vi "move.vi"(0 "x distance":dbl, 1 "y distance":dbl, 2 "z distance":dbl, 3 "button com":bool, 6 "handle":i32, 8 "halt":refnum<vi>, 9 "device ID":refnum<k1>, 10 "velocityZ":dbl, 11 "Encoder":T1, 12 "velocityX":dbl, 13 "velocityY":dbl, 14 "X Axis":u16(ring)=2 items=["X axis", "Y axis", "Z axis", "X axis rotation", "Y axis rotation", "Z axis rotation", "U axis", "V axis"], 15 "Y Axis":u16(ring)=1 items=["X axis", "Y axis", "Z axis", "X axis rotation", "Y axis rotation", "Z axis rotation", "U axis", "V axis"], 16 "Invert":bool, 17 "Invert 2":bool=TRUE, 18 "Invert 3":bool=TRUE, 19 "Z Axis":u16(ring)=4 items=["X axis", "Y axis", "Z axis", "X axis rotation", "Y axis rotation", "Z axis rotation", "U axis", "V axis"]) -> ()   [LabVIEW 2012]
uses:
  <vilib>/Utility/inputDevices.llb/joystickAcquire.vi
  MicroDrive.dll
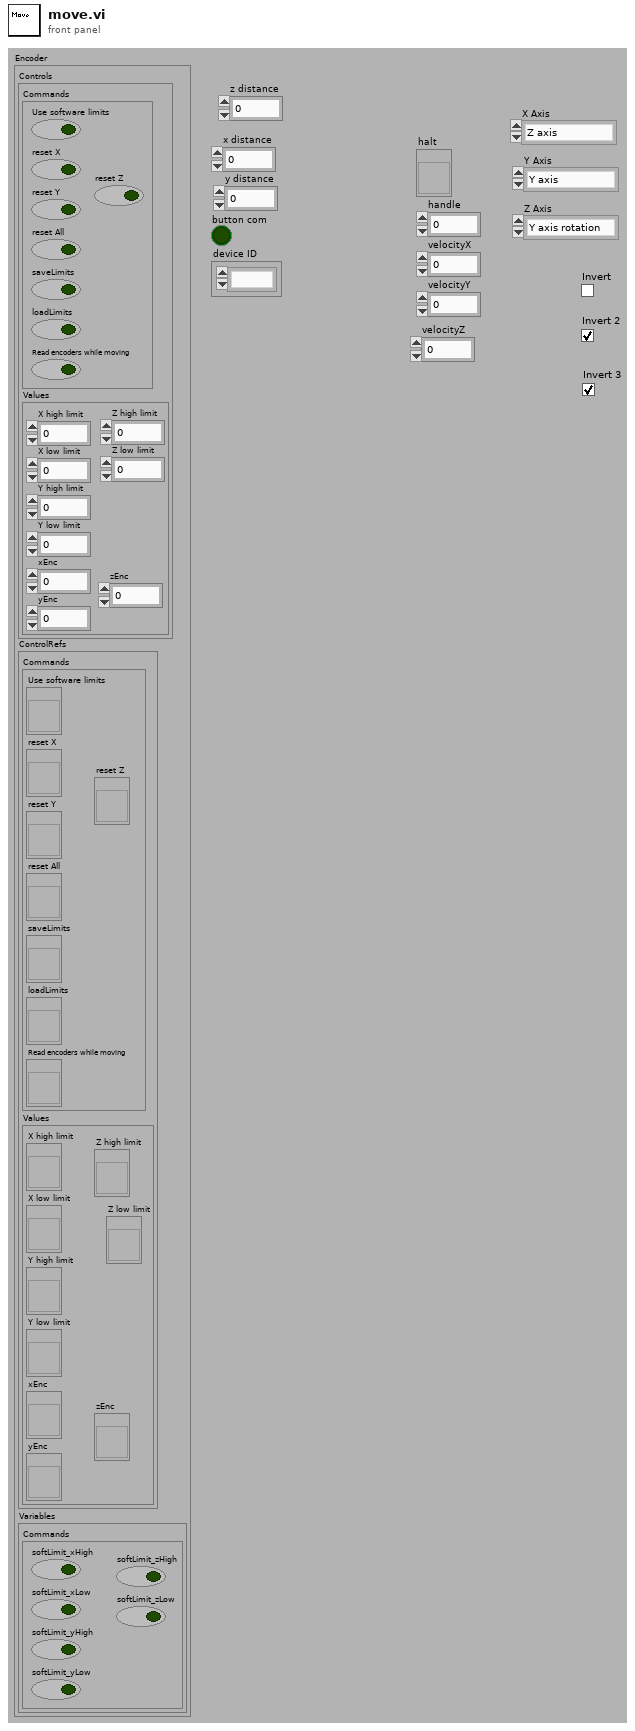
[diagram p1: front panel]
types:
  T1 = cluster{"Controls":cluster{"Commands":cluster{"Use software limits":bool, "reset X":bool, "reset Y":bool, "reset All":bool, "saveLimits":bool, "loadLimits":bool, "Read encoders while moving":bool, "reset Z":bool}, "Values":cluster{"X high limit":dbl, "X low limit":dbl, "Y high limit":dbl, "Y low limit":dbl, "xEnc":dbl, "yEnc":dbl, "Z low limit":dbl, "Z high limit":dbl, "zEnc":dbl}}, "ControlRefs":cluster{"Commands":cluster{"Use software limits":refnum<vi>, "reset X":refnum<vi>, "reset Y":refnum<vi>, "reset All":refnum<vi>, "saveLimits":refnum<vi>, "loadLimits":refnum<vi>, "Read encoders while moving":refnum<vi>, "reset Z":refnum<vi>}, "Values":cluster{"X high limit":refnum<vi>, "X low limit":refnum<vi>, "Y high limit":refnum<vi>, "Y low limit":refnum<vi>, "xEnc":refnum<vi>, "yEnc":refnum<vi>, "Z low limit":refnum<vi>, "Z high limit":refnum<vi>, "zEnc":refnum<vi>}}, "Variables":cluster{"Commands":cluster{"softLimit_xHigh":bool, "softLimit_xLow":bool, "softLimit_yHigh":bool, "softLimit_yLow":bool, "softLimit_zLow":bool, "softLimit_zHigh":bool}}}
  T2 = cluster{"xDistance":dbl, "yDistance":dbl, "xMove":bool, "yMove":bool, "zDistance":dbl, "zMove":bool}
  T3 = cluster{"Boolean array[0]":bool, "Boolean array[1]":bool, "Boolean array[2]":bool, "Boolean array[3]":bool, "Boolean array[4]":bool, "Boolean array[5]":bool, "Boolean array[6]":bool, "Boolean array[7]":bool, "Boolean array[8]":bool, "Boolean array[9]":bool, "Boolean array[10]":bool, "Boolean array[11]":bool, "Boolean array[12]":bool, "Boolean array[13]":bool, "Boolean array[14]":bool, "Boolean array[15]":bool}
  T4 = cluster{"X axis":i32, "Y axis":i32, "Z axis":i32, "X axis rotation":i32, "Y axis rotation":i32, "Z axis rotation":i32, "U axis":i32, "V axis":i32}
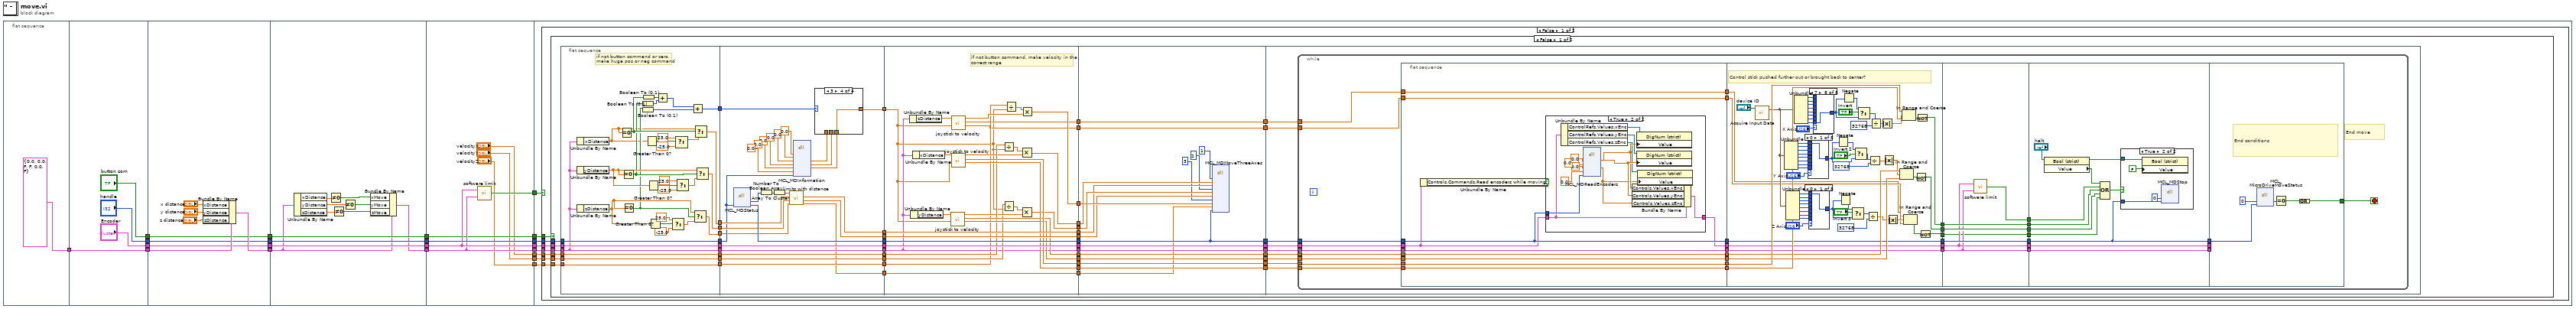
[diagram p0: block diagram]
diagram:
  n1 = flat-sequence {
    tunnel: [T2 {"xDistance"=0.0, "yDistance"=0.0, "xMove"=FALSE, "yMove"=FALSE, "zDistance"=0.0, "zMove"=FALSE}] -> w16
    tunnel: w16 -> [w26]
    tunnel: [w26] -> w15
    tunnel: ["Encoder"] -> w14
    tunnel: ["handle"] -> w13
    tunnel: ["button com"] -> w12
    tunnel: w15 -> [w34]
    tunnel: [w31] -> w21
    tunnel: w14 -> [w30]
    tunnel: w13 -> [w29]
    tunnel: w12 -> [w28]
    tunnel: [w30] -> w11
    tunnel: [w29] -> w10
    tunnel: [w28] -> w9
    tunnel: [w45] -> w7
    tunnel: [w43] -> w6
    tunnel: [w42] -> w5
    tunnel: [w44] -> w4
    tunnel: w9 -> [w44]
    tunnel: w10 -> [w45]
    tunnel: w11 -> [w43]
    tunnel: w21 -> [w38]
    tunnel: w7 -> [w53]
    tunnel: [w53] -> w20
    tunnel: w6 -> [w52]
    tunnel: [w52] -> w19
    tunnel: w5 -> [w51]
    tunnel: [w51] -> w18
    tunnel: [w50] -> w17
    tunnel: [w49] -> w8
    tunnel: w4 -> [w49]
    tunnel: ["velocityX"] -> w3
    tunnel: ["velocityY"] -> w2
    tunnel: ["velocityZ"] -> w1
    tunnel: w20 -> [w61]
    tunnel: w19 -> [w60]
    tunnel: w18 -> [w59]
    tunnel: w17 -> [w58]
    tunnel: w8 -> [w57]
    tunnel: w3 -> [w56]
    tunnel: w2 -> [w55]
    tunnel: w1 -> [w54]
    frame #0 {
    }
    frame #1 {
    }
    frame #2 {
      n2 = Bundle By Name(cluster=w34, "xDistance"="x distance", "yDistance"="y distance", "zDistance"="z distance") -> (w31:T2)
    }
    frame #3 {
      n3 = Unbundle By Name(w38) -> ("xDistance"=w41:dbl, "yDistance"=w37:dbl, "zDistance"=w36:dbl)
      n4 = Not Equal To 0?(x=w41) -> (x != 0?=w40:bool)
      n5 = Not Equal To 0?(x=w36) -> (x != 0?=w35:bool)
      n6 = Not Equal To 0?(x=w37) -> (x != 0?=w39:bool)
      n7 = Bundle By Name(cluster=w38, "xMove"=w40, "yMove"=w39, "zMove"=w35) -> (w42:T2)
    }
    frame #4 {
      n8 = call "software limit.vi"("variables"=w51, "Encoder"=w52) -> ("limited"=w50:bool)
    }
    frame #5 {
      n9 = case shown="False" w58 {
        tunnel: w57 -> [w68 _]
        tunnel: w61 -> [w67 _]
        tunnel: w60 -> [w66 _]
        tunnel: w59 -> [w65 _]
        tunnel: w56 -> [w64 _]
        tunnel: w55 -> [w63 _]
        tunnel: w54 -> [w62 _]
        frame False {
          n10 = case shown="False" w68 {
            tunnel: w67 -> [w118 w421]
            tunnel: w66 -> [w117 w420]
            tunnel: w65 -> [w112 w419]
            tunnel: w64 -> [w93 w415]
            tunnel: w63 -> [w91 w414]
            tunnel: w62 -> [w81 w413]
            frame False {
              n11 = flat-sequence {
                tunnel: w117 -> [w149]
                tunnel: w118 -> [w150]
                tunnel: [w150] -> w116
                tunnel: [w140] -> w115
                tunnel: [w139] -> w114
                tunnel: [w149] -> w113
                tunnel: w112 -> [w136]
                tunnel: [w136] -> w111
                tunnel: [w138] -> w94
                tunnel: w93 -> [w138]
                tunnel: [w137] -> w92
                tunnel: w91 -> [w137]
                tunnel: w81 -> [w129]
                tunnel: [w132] -> w80
                tunnel: [w129] -> w79
                tunnel: [w119] -> w70
                tunnel: [w175] -> w110
                tunnel: [w166] -> w108
                tunnel: [w165] -> w106
                tunnel: [w171] -> w104
                tunnel: w116 -> [w164]
                tunnel: w115 -> [w173]
                tunnel: w114 -> [w172]
                tunnel: w113 -> [w171]
                tunnel: [w170] -> w102
                tunnel: w111 -> [w170]
                tunnel: w94 -> [w169]
                tunnel: w92 -> [w168]
                tunnel: [w169] -> w90
                tunnel: [w168] -> w89
                tunnel: w80 -> [w152]
                tunnel: w79 -> [w167]
                tunnel: [w167] -> w78
                tunnel: [w151] -> w76
                tunnel: w70 -> [w157]
                tunnel: [w153] -> w69
                tunnel: w110 -> [w209]
                tunnel: [w209] -> w109
                tunnel: w108 -> [w208]
                tunnel: [w208] -> w107
                tunnel: w106 -> [w207]
                tunnel: [w207] -> w105
                tunnel: w104 -> [w206]
                tunnel: [w206] -> w103
                tunnel: w102 -> [w192]
                tunnel: [w192] -> w101
                tunnel: [w197] -> w100
                tunnel: [w203] -> w99
                tunnel: [w202] -> w98
                tunnel: [w194] -> w97
                tunnel: [w201] -> w96
                tunnel: [w200] -> w95
                tunnel: w90 -> [w199]
                tunnel: w89 -> [w193]
                tunnel: w78 -> [w186]
                tunnel: [w189] -> w77
                tunnel: w76 -> [w185]
                tunnel: [w185] -> w75
                tunnel: [w184] -> w73
                tunnel: [w183] -> w71
                tunnel: w69 -> [w182]
                tunnel: [w227] -> w88
                tunnel: [w226] -> w87
                tunnel: [w225] -> w86
                tunnel: [w224] -> w85
                tunnel: [w223] -> w84
                tunnel: [w221] -> w83
                tunnel: [w222] -> w82
                tunnel: w95 -> [w224]
                tunnel: w96 -> [w225]
                tunnel: w97 -> [w217]
                tunnel: w98 -> [w226]
                tunnel: w99 -> [w227]
                tunnel: w100 -> [w218]
                tunnel: w101 -> [w222]
                tunnel: w103 -> [w223]
                tunnel: w105 -> [w214]
                tunnel: w107 -> [w215]
                tunnel: w109 -> [w221]
                tunnel: w77 -> [w216]
                tunnel: w75 -> [w213]
                tunnel: [w220] -> w74
                tunnel: w73 -> [w220]
                tunnel: [w219] -> w72
                tunnel: w71 -> [w219]
                tunnel: w88 -> [w236]
                tunnel: w87 -> [w235]
                tunnel: w86 -> [w234]
                tunnel: w85 -> [w233]
                tunnel: w84 -> [w232]
                tunnel: w83 -> [w231]
                tunnel: w82 -> [w230]
                tunnel: w74 -> [w229]
                tunnel: w72 -> [w228]
                frame #0 {
                  # "if not button command or zero,\nmake huge pos or neg command"
                  n12 = Unbundle By Name(w136) -> ("yDistance"=w127:dbl)
                  n13 = Unbundle By Name(w136) -> ("xDistance"=w120:dbl)
                  n14 = Unbundle By Name(w136) -> ("zDistance"=w130:dbl)
                  n15 = Equal To 0?(x=w120) -> (x = 0?=w128:bool)
                  n16 = Equal To 0?(x=w127) -> (x = 0?=w122:bool)
                  n17 = Equal To 0?(x=w130) -> (x = 0?=w121:bool)
                  n18 = Boolean To (0,1)(Boolean=w122) -> (0, 1=w125:i16)
                  n19 = Boolean To (0,1)(Boolean=w121) -> (0, 1=w124:i16)
                  n20 = Boolean To (0,1)(Boolean=w128) -> (0, 1=w126:i16)
                  n21 = Greater Than 0?(x=w120) -> (x > 0?=w147:bool)
                  n22 = Greater Than 0?(x=w127) -> (x > 0?=w143:bool)
                  n23 = Greater Than 0?(x=w130) -> (x > 0?=w135:bool)
                  n24 = Add(x=w126, y=w125) -> (x+y=w123:i16)
                  n25 = Select(t=25.0, s=w135, f=-25.0) -> (s? t:f=w131:dbl)
                  n26 = Select(t=25.0, s=w147, f=-25.0) -> (s? t:f=w148:dbl)
                  n27 = Select(t=25.0, s=w143, f=-25.0) -> (s? t:f=w144:dbl)
                  n28 = Add(x=w123, y=w124) -> (x+y=w119:i16)
                  n29 = Select(t=w130, s=w121, f=w131) -> (s? t:f=w132:dbl)
                  n30 = Select(t=w120, s=w128, f=w148) -> (s? t:f=w140:dbl)
                  n31 = Select(t=w127, s=w122, f=w144) -> (s? t:f=w139:dbl)
                }
                frame #1 {
                  n32 = dll-call lib="C:/Users/Labview/Desktop/SRR/MicroDrive_x64/Labview Examples/MicroDrive.dll" fn="MCL_MDStatus"("handle"=w164) -> ("status"=w177:u16, "handle"=w175:i32)  [unwired: 3 in, 4 out]
                  n33 = Number To Boolean Array(number=w177) -> (Boolean array=w176:bool[])
                  n34 = Array To Cluster(array=w176) -> (cluster=w174:T3)
                  n35 = call "limits with distance.vi"("distanceM3"=w152, "distanceM2"=w172, "distanceM1"=w173, "cluster"=w174) -> ("M3 Distance"=w151:dbl, "M2 Distance"=w165:dbl, "M1 Distance"=w166:dbl)  [unwired: 1 in, 4 out]
                  n36 = dll-call lib="C:/Users/Labview/Desktop/SRR/MicroDrive_x64/Labview Examples/MicroDrive.dll" fn="MCL_MDInformation"("encoderResolution"=0.0 ("t"), "stepSize"=0.0 ("t"), "maxVelocity"=0.0 ("t"), "maxVelocityTwoAxis"=0.0 ("t"), "maxVelocityThreeAxis"=0.0 ("t"), "minVelocity"=0.0 ("t"), "handle"=w164) -> ("maxVelocity"=w156:dbl, "maxVelocityTwoAxis"=w155:dbl, "maxVelocityThreeAxis"=w154:dbl)  [unwired: 4 in, 6 out]
                  n37 = case shown="3" w157 {
                    tunnel: w156 -> [w178 w179 _ _]
                    tunnel: w155 -> [_ _ w180 _]
                    tunnel: w154 -> [_ _ _ w181]
                    tunnel: [w178 w179 w180 w181] -> w153
                    frame 0, Default {
                    }
                    frame 1 {
                    }
                    frame 2 {
                    }
                    frame 3 {
                    }
                  }
                }
                frame #2 {
                  # "if not button command, make velocity in the\ncorrect range"
                  n38 = Unbundle By Name(w192) -> ("zDistance"=w191:dbl)
                  n39 = Unbundle By Name(w192) -> ("yDistance"=w205:dbl)
                  n40 = Unbundle By Name(w192) -> ("xDistance"=w204:dbl)
                  n41 = call "joystick to velocity.vi"("max velocity"=w182, "joystick main"=w205) -> ("lower bound"=w200:dbl, "upper bound"=w201:dbl, "Velocity"=w195:dbl)  [unwired: 2 in, 5 out]
                  n42 = call "joystick to velocity.vi"("max velocity"=w182, "joystick main"=w191) -> ("lower bound"=w183:dbl, "upper bound"=w184:dbl, "Velocity"=w187:dbl)  [unwired: 2 in, 5 out]
                  n43 = call "joystick to velocity.vi"("max velocity"=w182, "joystick main"=w204) -> ("lower bound"=w202:dbl, "upper bound"=w203:dbl, "Velocity"=w198:dbl)  [unwired: 2 in, 5 out]
                  n44 = Divide(x=w199, y=w182) -> (x/y=w190:dbl)
                  n45 = Divide(x=w193, y=w182) -> (x/y=w196:dbl)
                  n46 = Divide(x=w186, y=w182) -> (x/y=w188:dbl)
                  n47 = Multiply(x=w190, y=w198) -> (x*y=w197:dbl)
                  n48 = Multiply(x=w196, y=w195) -> (x*y=w194:dbl)
                  n49 = Multiply(x=w188, y=w187) -> (x*y=w189:dbl)
                }
                frame #3 {
                  n50 = dll-call lib="C:/Users/Labview/Desktop/SRR/MicroDrive_x64/Labview Examples/MicroDrive.dll" fn="MCL_MDMoveThreeAxes"("axis1"=1 ("rounding-X"), "Velocity-1"=w218, "distance-1"=w215, "axis2"=2 ("rounding-X"), "Velocity-2"=w217, "distance-2"=w214, "axis3"=3 ("rounding-X"), "Velocity-3"=w216, "Distance-3"=w213, "handle"=w221) -> ()  [unwired: 14 in, 2 out]
                }
                frame #4 {
                  n51 = while {
                    tunnel: w236 -> [w270]
                    tunnel: w235 -> [w269]
                    tunnel: w234 -> [w268]
                    tunnel: w233 -> [w267]
                    tunnel: w232 -> [w266]
                    tunnel: w231 -> [w265]
                    tunnel: w230 -> [w262]
                    tunnel: w229 -> [w240]
                    tunnel: w228 -> [w238]
                    stop <- w271 stop-if-true
                    # "End move"
                    n52 = flat-sequence {
                      tunnel: w262 -> [w276]
                      tunnel: w265 -> [w278]
                      tunnel: w266 -> [w275]
                      tunnel: w267 -> [w279]
                      tunnel: w268 -> [w280]
                      tunnel: w269 -> [w281]
                      tunnel: w270 -> [w282]
                      tunnel: [w282] -> w249
                      tunnel: [w281] -> w248
                      tunnel: [w280] -> w247
                      tunnel: [w279] -> w246
                      tunnel: [w277] -> w245
                      tunnel: [w278] -> w244
                      tunnel: [w276] -> w243
                      tunnel: w240 -> [w273]
                      tunnel: [w273] -> w239
                      tunnel: w238 -> [w272]
                      tunnel: [w272] -> w237
                      tunnel: [w321] -> w260
                      tunnel: [w324] -> w258
                      tunnel: [w339] -> w256
                      tunnel: [w322] -> w254
                      tunnel: [w320] -> w252
                      tunnel: w249 -> [w342]
                      tunnel: w248 -> [w341]
                      tunnel: w247 -> [w329]
                      tunnel: w246 -> [w340]
                      tunnel: w245 -> [w322]
                      tunnel: w244 -> [w321]
                      tunnel: w243 -> [w320]
                      tunnel: [w307] -> w242
                      tunnel: w239 -> [w297]
                      tunnel: w237 -> [w298]
                      tunnel: w260 -> [w392]
                      tunnel: [w392] -> w259
                      tunnel: w258 -> [w391]
                      tunnel: [w391] -> w257
                      tunnel: w256 -> [w390]
                      tunnel: [w390] -> w255
                      tunnel: w254 -> [w388]
                      tunnel: [w388] -> w253
                      tunnel: w252 -> [w389]
                      tunnel: [w389] -> w251
                      tunnel: [w387] -> w250
                      tunnel: w242 -> [w386]
                      tunnel: [w386] -> w241
                      tunnel: [w403] -> w264
                      tunnel: [w401] -> w263
                      tunnel: [w402] -> w261
                      tunnel: w250 -> [w394]
                      tunnel: w251 -> [w402]
                      tunnel: w253 -> [w401]
                      tunnel: w255 -> [w395]
                      tunnel: w257 -> [w396]
                      tunnel: w259 -> [w403]
                      tunnel: w241 -> [w397]
                      tunnel: [w408] -> w271
                      tunnel: w261 -> [_]
                      tunnel: w263 -> [_]
                      tunnel: w264 -> [w411]
                      frame #0 {
                        n53 = Unbundle By Name(w275) -> ("Controls.Commands.Read encoders while moving"=w274:bool)
                        n54 = case shown="True" w274 {
                          tunnel: w278 -> [_ w292]
                          tunnel: [w283 w291] -> w277
                          tunnel: w275 -> [w283 w290]
                          frame False {
                          }
                          frame True {
                            n55 = Unbundle By Name(w290) -> ("ControlRefs.Values.xEnc"=w294:refnum<vi>, "ControlRefs.Values.yEnc"=w293:refnum<vi>, "ControlRefs.Values.zEnc"=w286:refnum<vi>)
                            n56 = dll-call lib="C:/Users/Labview/Desktop/SRR/MicroDrive_x64/Labview Examples/MicroDrive.dll" fn="MCL_MDReadEncoders"("e1"=0.0 ("x enc"), "e2"=0.0 ("y enc"), "e3"=0.0 ("z enc"), "e4"=0.0 ("z enc"), "handle"=w292) -> ("e1"=w287:dbl, "e2"=w288:dbl, "e3"=w285:dbl)  [unwired: 4 in, 4 out]
                            n57 = Bundle By Name(cluster=w290, "Controls.Values.xEnc"=w287, "Controls.Values.yEnc"=w288, "Controls.Values.zEnc"=w285) -> (w291:T1)
                            n58 = property class="DigNum (strict)"(reference=w294, "Value"=w287) -> ()  [unwired: 1 in, 2 out]
                            n59 = property class="DigNum (strict)"(reference=w293, "Value"=w288) -> ()  [unwired: 1 in, 2 out]
                            n60 = property class="DigNum (strict)"(reference=w286, "Value"=w285) -> ()  [unwired: 1 in, 2 out]
                          }
                        }
                      }
                      frame #1 {
                        # "Control stick pushed further out or brought back to center?"
                        n61 = call-poly <vilib>:"Acquire Input Data.vi"("device ID"="device ID") -> ("axis info"=w317:T4)  [unwired: 2 in, 16 out]
                        n62 = Unbundle(w317) -> ("X axis"=w331:i32, "Y axis"=w332:i32, "Z axis"=w333:i32, "X axis rotation"=w334:i32, "Y axis rotation"=w335:i32, "Z axis rotation"=w336:i32, "U axis"=w337:i32, "V axis"=w338:i32)
                        n63 = Unbundle(w317) -> ("X axis"=w316:i32, "Y axis"=w315:i32, "Z axis"=w314:i32, "X axis rotation"=w313:i32, "Y axis rotation"=w312:i32, "Z axis rotation"=w311:i32, "U axis"=w310:i32, "V axis"=w309:i32)
                        n64 = Unbundle(w317) -> ("X axis"=w345:i32, "Y axis"=w346:i32, "Z axis"=w347:i32, "X axis rotation"=w348:i32, "Y axis rotation"=w349:i32, "Z axis rotation"=w350:i32, "U axis"=w351:i32, "V axis"=w352:i32)
                        n65 = case shown="0" "Y Axis" {
                          tunnel: w331 -> [w370 _ _ _ _ _ _ _]
                          tunnel: w332 -> [_ w371 _ _ _ _ _ _]
                          tunnel: w333 -> [_ _ w372 _ _ _ _ _]
                          tunnel: w334 -> [_ _ _ w373 _ _ _ _]
                          tunnel: w335 -> [_ _ _ _ w374 _ _ _]
                          tunnel: w336 -> [_ _ _ _ _ w375 _ _]
                          tunnel: w337 -> [_ _ _ _ _ _ w376 _]
                          tunnel: w338 -> [_ _ _ _ _ _ _ w377]
                          tunnel: [w370 w371 w372 w373 w374 w375 w376 w377] -> w330
                          frame 0 {
                          }
                          frame 1 {
                          }
                          frame 2, Default {
                          }
                          frame 3 {
                          }
                          frame 4 {
                          }
                          frame 5 {
                          }
                          frame 6 {
                          }
                          frame 7 {
                          }
                        }
                        n66 = case shown="0" "Z Axis" {
                          tunnel: w316 -> [w362 _ _ _ _ _ _ _]
                          tunnel: w315 -> [_ w363 _ _ _ _ _ _]
                          tunnel: w314 -> [_ _ w364 _ _ _ _ _]
                          tunnel: w313 -> [_ _ _ w365 _ _ _ _]
                          tunnel: w312 -> [_ _ _ _ w366 _ _ _]
                          tunnel: w311 -> [_ _ _ _ _ w367 _ _]
                          tunnel: w310 -> [_ _ _ _ _ _ w368 _]
                          tunnel: w309 -> [_ _ _ _ _ _ _ w369]
                          tunnel: [w362 w363 w364 w365 w366 w367 w368 w369] -> w304
                          frame 0 {
                          }
                          frame 1 {
                          }
                          frame 2, Default {
                          }
                          frame 3 {
                          }
                          frame 4 {
                          }
                          frame 5 {
                          }
                          frame 6 {
                          }
                          frame 7 {
                          }
                        }
                        n67 = case shown="7" "X Axis" {
                          tunnel: w345 -> [w378 _ _ _ _ _ _ _]
                          tunnel: w346 -> [_ w379 _ _ _ _ _ _]
                          tunnel: w347 -> [_ _ w380 _ _ _ _ _]
                          tunnel: w348 -> [_ _ _ w381 _ _ _ _]
                          tunnel: w349 -> [_ _ _ _ w382 _ _ _]
                          tunnel: w350 -> [_ _ _ _ _ w383 _ _]
                          tunnel: w351 -> [_ _ _ _ _ _ w384 _]
                          tunnel: w352 -> [_ _ _ _ _ _ _ w385]
                          tunnel: [w378 w379 w380 w381 w382 w383 w384 w385] -> w358
                          frame 0 {
                          }
                          frame 1 {
                          }
                          frame 2, Default {
                          }
                          frame 3 {
                          }
                          frame 4 {
                          }
                          frame 5 {
                          }
                          frame 6 {
                          }
                          frame 7 {
                          }
                        }
                        n68 = Negate(x=w330) -> (-x=w355:i32)
                        n69 = Negate(x=w304) -> (-x=w305:i32)
                        n70 = Negate(x=w358) -> (-x=w357:i32)
                        n71 = Select(t=w305, s="Invert 3", f=w304) -> (s? t:f=w302:i32)
                        n72 = Select(t=w355, s="Invert 2", f=w330) -> (s? t:f=w360:i32)
                        n73 = Select(t=w357, s="Invert", f=w358) -> (s? t:f=w359:i32)
                        n74 = Divide(x=w302, y=32768) -> (x/y=w300:dbl)
                        n75 = Divide(x=w360, y=32768) -> (x/y=w343:dbl)
                        n76 = Divide(x=w359, y=32768) -> (x/y=w328:dbl)
                        n77 = Absolute Value(x=w328) -> (abs(x)=w327:dbl)
                        n78 = Absolute Value(x=w343) -> (abs(x)=w326:dbl)
                        n79 = Absolute Value(x=w300) -> (abs(x)=w299:dbl)
                        n80 = In Range and Coerce(upper limit=w329, x=w326, lower limit=w340) -> (In Range?=w325:bool)  [unwired: 1 out]
                        n81 = In Range and Coerce(upper limit=w342, x=w327, lower limit=w341) -> (In Range?=w323:bool)  [unwired: 1 out]
                        n82 = In Range and Coerce(upper limit=w297, x=w299, lower limit=w298) -> (In Range?=w306:bool)  [unwired: 1 out]
                        n83 = Not(x=w325) -> (.not. x?=w324:bool)
                        n84 = Not(x=w323) -> (.not. x?=w339:bool)
                        n85 = Not(x=w306) -> (.not. x?=w307:bool)
                      }
                      frame #2 {
                        n86 = call "software limit.vi"("variables"=w389, "Encoder"=w388) -> ("limited"=w387:bool)
                      }
                      frame #3 {
                        n87 = property on="Property Node" class="Bool (strict)"(reference="halt") -> (reference out=w399:refnum<vi>, "Value"=w393:bool)  [unwired: 1 in, 1 out]
                        n88 = Compound Arithmetic op=OR(w393, w394, w395, w396, w397) -> (w398:bool)
                        n89 = case shown="True" w398 {
                          tunnel: w403 -> [_ w405]
                          tunnel: w399 -> [_ w406]
                          frame False {
                          }
                          frame True {
                            n90 = property on="Property Node" class="Bool (strict)"(reference=w406, "Value"=FALSE) -> ()  [unwired: 1 in, 2 out]
                            n91 = dll-call lib="C:/Users/Labview/Desktop/SRR/MicroDrive_x64/Labview Examples/MicroDrive.dll" fn="MCL_MDStop"("status"=u16 0, "handle"=w405) -> ()  [unwired: 4 in, 4 out]
                          }
                        }
                      }
                      frame #4 {
                        # "End conditions"
                        n92 = dll-call lib="C:/Users/Labview/Desktop/SRR/MicroDrive_x64/Labview Examples/MicroDrive.dll" fn="MCL_MicroDriveMoveStatus"("isMoving"=0 ("axis"), "handle"=w411) -> ("isMoving"=w410:i32)  [unwired: 4 in, 3 out]
                        n93 = Equal To 0?(x=w410) -> (x = 0?=w409:bool)
                        n94 = Compound Arithmetic op=OR(w409) -> (w408:bool)
                      }
                    }
                  }
                }
              }
            }
            frame True {
              n95 = flat-sequence {
                tunnel: [w428] -> w418
                tunnel: [w433] -> w417
                tunnel: [w432] -> w416
                tunnel: w421 -> [w428]
                tunnel: w420 -> [w433]
                tunnel: w419 -> [w432]
                tunnel: w415 -> [w427]
                tunnel: w414 -> [w426]
                tunnel: w413 -> [w425]
                tunnel: w418 -> [w436]
                tunnel: w417 -> [w435]
                tunnel: w416 -> [w434]
                frame #0 {
                  n96 = Unbundle By Name(w432) -> ("xDistance"=w431:dbl, "yDistance"=w430:dbl, "zDistance"=w429:dbl)
                  n97 = dll-call lib="C:/Users/Labview/Desktop/SRR/MicroDrive_x64/Labview Examples/MicroDrive.dll" fn="MCL_MDMoveThreeAxes"("axis1"=1 ("RoundingX"), "Velocity1"=w427, "Distance1"=w431, "axis2"=2 ("RoundingX"), "Velocity2"=w426, "Distance2"=w430, "axis3"=3 ("RoundingX"), "Velocity3"=w425, "Distance3"=w429, "handle"=w428) -> ()  [unwired: 14 in, 2 out]
                }
                frame #1 {
                  n98 = while {
                    tunnel: w436 -> [w448]
                    tunnel: w435 -> [w446]
                    tunnel: w434 -> [w441]
                    stop <- w447 stop-if-true
                    n99 = flat-sequence {
                      tunnel: w448 -> [w450]
                      tunnel: [w450] -> w442
                      tunnel: w446 -> [w451]
                      tunnel: [w449] -> w443
                      tunnel: w441 -> [w453]
                      tunnel: [w453] -> w440
                      tunnel: [w470] -> w439
                      tunnel: [w471] -> w438
                      tunnel: [w468] -> w437
                      tunnel: w443 -> [w470]
                      tunnel: w442 -> [w471]
                      tunnel: w440 -> [w469]
                      tunnel: [w479] -> w445
                      tunnel: [w472] -> w444
                      tunnel: w439 -> [w472]
                      tunnel: w438 -> [w477]
                      tunnel: w437 -> [w473]
                      tunnel: w445 -> [w489]
                      tunnel: [w486] -> w447
                      tunnel: w444 -> [w488]
                      tunnel: [w488] -> _
                      frame #0 {
                        n100 = Unbundle By Name(w451) -> ("Controls.Commands.Read encoders while moving"=w452:bool)
                        n101 = case shown="True" w452 {
                          tunnel: w450 -> [_ w463]
                          tunnel: [w454 w462] -> w449
                          tunnel: w451 -> [w454 w458]
                          frame False {
                          }
                          frame True {
                            n102 = Unbundle By Name(w458) -> ("ControlRefs.Values.xEnc"=w465:refnum<vi>, "ControlRefs.Values.yEnc"=w464:refnum<vi>, "ControlRefs.Values.zEnc"=w457:refnum<vi>)
                            n103 = dll-call lib="C:/Users/Labview/Desktop/SRR/MicroDrive_x64/Labview Examples/MicroDrive.dll" fn="MCL_MDReadEncoders"("e1"=0.0 ("x enc"), "e2"=0.0 ("y enc"), "e3"=0.0 ("z enc"), "e4"=0.0 ("y enc"), "handle"=w463) -> ("e1"=w460:dbl, "e2"=w459:dbl, "e3"=w456:dbl)  [unwired: 4 in, 4 out]
                            n104 = Bundle By Name(cluster=w458, "Controls.Values.xEnc"=w460, "Controls.Values.yEnc"=w459, "Controls.Values.zEnc"=w456) -> (w462:T1)
                            n105 = property class="DigNum (strict)"(reference=w465, "Value"=w460) -> ()  [unwired: 1 in, 2 out]
                            n106 = property class="DigNum (strict)"(reference=w464, "Value"=w459) -> ()  [unwired: 1 in, 2 out]
                            n107 = property class="DigNum (strict)"(reference=w457, "Value"=w456) -> ()  [unwired: 1 in, 2 out]
                          }
                        }
                      }
                      frame #1 {
                        n108 = call "software limit.vi"("variables"=w469, "Encoder"=w470) -> ("limited"=w468:bool)
                      }
                      frame #2 {
                        n109 = local read "halt"() -> (w476:refnum<vi>)
                        n110 = property on="Property Node" class="Bool (strict)"(reference=w476) -> (reference out=w478:refnum<vi>, "Value"=w475:bool)  [unwired: 1 in, 1 out]
                        n111 = Compound Arithmetic op=OR(w475, w473) -> (w474:bool)
                        n112 = case shown="True" w474 {
                          tunnel: w477 -> [w480 w481]
                          tunnel: [w480 w482] -> w479
                          tunnel: w478 -> [_ w484]
                          frame False {
                          }
                          frame True {
                            n113 = property on="Property Node" class="Bool (strict)"(reference=w484, "Value"=FALSE) -> ()  [unwired: 1 in, 2 out]
                            n114 = dll-call lib="C:/Users/Labview/Desktop/SRR/MicroDrive_x64/Labview Examples/MicroDrive.dll" fn="MCL_MDStop"("status"=u16 0, "handle"=w481) -> ("handle"=w482:i32)  [unwired: 3 in, 4 out]
                          }
                        }
                      }
                      frame #3 {
                        n115 = dll-call lib="C:/Users/Labview/Desktop/SRR/MicroDrive_x64/Labview Examples/MicroDrive.dll" fn="MCL_MicroDriveMoveStatus"("isMoving"=0 ("axis"), "handle"=w489) -> ("isMoving"=w490:i32)  [unwired: 4 in, 3 out]
                        n116 = Equal To 0?(x=w490) -> (x = 0?=w487:bool)
                        n117 = Compound Arithmetic op=OR(w487) -> (w486:bool)
                      }
                    }
                  }
                }
              }
            }
          }
        }
        frame True {
        }
      }
    }
  }
